vi "Close Cell Refnum.vi"(1 "References":T3, 11 "error in (no error)":errorcluster) -> (15 "error out":errorcluster)   [LabVIEW 2012]
doc: "Version 1.0\nDeveloped by Jean-Marc Simard\nCopyright © 2010, Exaprom Inc.\nAll rights reserved.\nLicense: BSD\n\nWith iTextSharp 4.1.6 (http://itextsharp.sourceforge.net)\nunder Mozilla Public License Version 1.1\n(http://www.mozilla.org/MPL/MPL-1.1.html)"
uses:
  Controls/Cell Generic Format without Font.ctl
  C:/Users/MaxCorp/Documents/TopPerm - Base/DLL/itextsharp.dll
  DLL/itextsharp.dll
  Controls/Cell Border.ctl
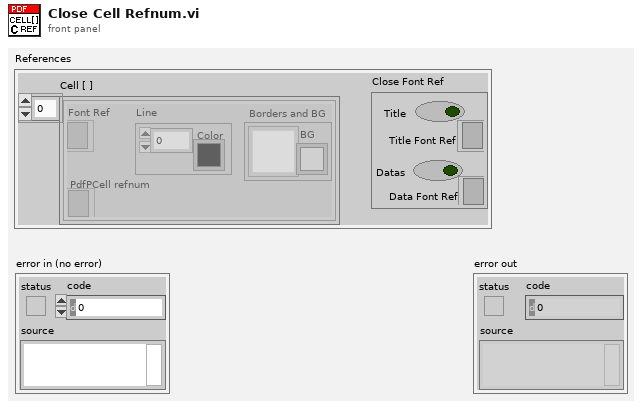
[diagram p1: front panel]
types:
  T1 = typedef "Cell Generic Format without Font.ctl" = cluster{"Font Ref":refnum<k24>, "Line":cluster{"Thickness":sgl, "Color":u32}, "Borders and BG":cluster{"Cell Border":T2, "BG":u32}, "PdfPCell refnum":refnum<k24>}
  T2 = typedef "Cell Border.ctl" = u16
  T3 = cluster{"Cell [ ]":T1[], "Close Font Ref":cluster{"Title":bool, "Title Font Ref":refnum<k24>, "Datas":bool, "Data Font Ref":refnum<k24>}}
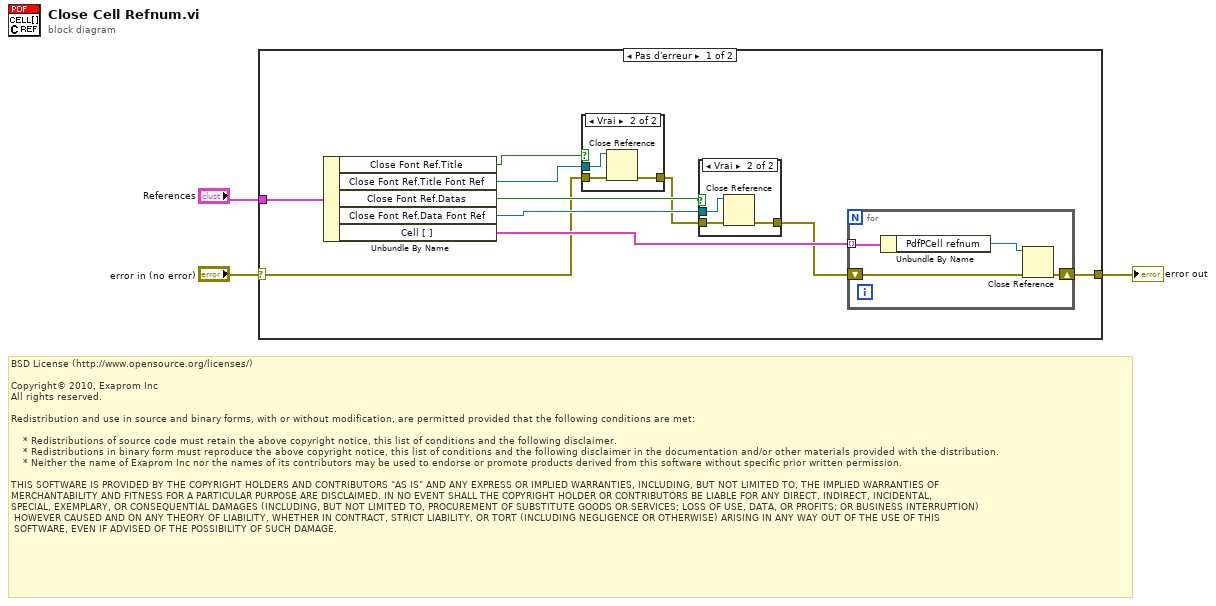
[diagram p0: block diagram]
diagram:
  # "BSD License (http://www.opensource.org/licenses/)\n\nCopyright© 2010, Exaprom Inc\nAll rights reserved.\n\nRedistribution and use in source and binary forms, with or without modification, are permitted provided that the following conditions are met:\n\n    * Redistributions of source code must retain the above copyright notice, this list of conditions and the following disclaimer.\n    * Redistributions in binary form must reproduce the above copyright notice, this list of conditions and the following disclaimer in the documentation and/or other materials provided with the distribution.\n    * Neither the name of Exaprom Inc nor the names of its contributors may be used to endorse or promote products derived from this software without specific prior written permission.\n\nTHIS SOFTWARE IS PROVIDED BY THE COPYRIGHT HOLDERS AND CONTRIBUTORS \"AS IS\" AND ANY EXPRESS OR IMPLIED WARRANTIES, INCLUDING, BUT NOT LIMITED TO, THE IMPLIED WARRANTIES OF \nMERCHANTABILITY AND FITNESS FOR A PARTICULAR PURPOSE ARE DISCLAIMED. IN NO EVENT SHALL THE COPYRIGHT HOLDER OR CONTRIBUTORS BE LIABLE FOR ANY DIRECT, INDIRECT, INCIDENTAL,\nSPECIAL, EXEMPLARY, OR CONSEQUENTIAL DAMAGES (INCLUDING, BUT NOT LIMITED TO, PROCUREMENT OF SUBSTITUTE GOODS OR SERVICES; LOSS OF USE, DATA, OR PROFITS; OR BUSINESS INTERRUPTION)\n HOWEVER CAUSED AND ON ANY THEORY OF LIABILITY, WHETHER IN CONTRACT, STRICT LIABILITY, OR TORT (INCLUDING NEGLIGENCE OR OTHERWISE) ARISING IN ANY WAY OUT OF THE USE OF THIS\n SOFTWARE, EVEN IF ADVISED OF THE POSSIBILITY OF SUCH DAMAGE."
  n1 = case shown="Pas d'erreur" "error in (no error)" {
    selector: "error in (no error)" -> [w5 w26]
    tunnel: [w4 w26] -> w3
    tunnel: "References" -> [w13 _]
    frame No Error {
      n2 = Unbundle By Name(w13) -> ("Close Font Ref.Title"=w12:bool, "Close Font Ref.Title Font Ref"=w11:refnum<k24>, "Close Font Ref.Datas"=w10:bool, "Close Font Ref.Data Font Ref"=w9:refnum<k24>, "Cell [ ]"=w7:T1[])
      n3 = case shown="Vrai" w12 {
        tunnel: w11 -> [_ w25]
        tunnel: w5 -> [w22 w24]
        tunnel: [w22 w23] -> w8
        frame False {
        }
        frame True {
          n4 = Close Reference(reference=w25, error in (no error)=w24) -> (error out=w23:errorcluster)
        }
      }
      n5 = case shown="Vrai" w10 {
        tunnel: w9 -> [_ w21]
        tunnel: w8 -> [w18 w20]
        tunnel: [w18 w19] -> w6
        frame False {
        }
        frame True {
          n6 = Close Reference(reference=w21, error in (no error)=w20) -> (error out=w19:errorcluster)
        }
      }
      n7 = for {
        tunnel: w7 -> [w17] mode=indexing
        shift-right: [w14] -> w4
        shift-left: w6 -> [w15]
        n8 = Unbundle By Name(w17) -> ("PdfPCell refnum"=w16:refnum<k24>)
        n9 = Close Reference(reference=w16, error in (no error)=w15) -> (error out=w14:errorcluster)
      }
    }
    frame Error {
    }
  }
  "error out" <- w3
